vi "xyz-fluor_localisation.vi"(4 "Positive angle":dbl, 5 "Gy":dbl[][](array[numeric]), 6 "Gthr":dbl[][](array[numeric]), 7 "Gx":dbl[][](array[numeric]), 8 "R":dbl, 9 "weights":dbl[](array[numeric]), 10 "B points":dbl[][](array[numeric])=[[5.0, 3.0], [6.0, 6.0]], 11 "A points":dbl[][](array[numeric])=[[0.0, 1.0], [2.0, 3.0]]) -> (3 "XYZ":dbl[](array[numeric]))   [LabVIEW 2015]
doc: "INPUT\nR - radius of the window (should be >0.5)\nGx,Gy - horizontal and vertical local gradient images\nGthr - thresholded magnitude of local gradients (if not wired will be calculated from Gx,Gy)\nA points - 2xN array of first points that define lines\nB points - 2xN array of second points that define lines\nw - weights (1D array)\nPositive angle - angle in degrees that defines orientation of the image of the particle which corresponds to positive z-value\n\nOUTPUT\nXYZ - x,y position of the particle in pixels (for original image), z-value\n\nThis vi calculates XYZ position of the fluorescent particle in astigmatism based microscopy. XY is found as a least square intersection point of gradient lines. The image of local gradients (Gthr) is splitted into 4 parts: TOP, LEFT, BOTTOM, RIGHT, relative to the particle center (cx,cy). The least-square intersection of all gradient lines (Gx, Gy) is calculated for each part. These centers are forming two lines: TOP-BOTTOM and LEFT-RIGHT, which are called axes (similar to ellipses axes). The major of two axes represents the magnitude of the z-value. The sign of the z-value is determined according to the angPos value which should correspond to the position of the long axis of the elliptical image of the particle. angPos is not required to be accurate, however, setting it to ~45 degrees off the real angle will create sporadic change in the sign and, therefore, in z-value.\n\nAuthor: Anatolii Kashchuk"
panel:
  out "center":dbl[][](array[numeric])
  # "This vi finds centroid and z-value from the image of a particle\n\nAuthor: Anatolii Kashchuk"
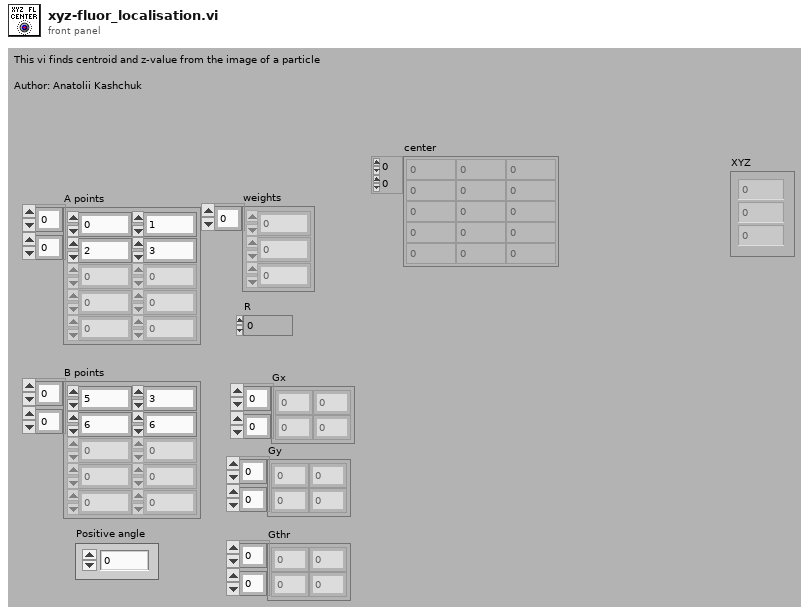
[diagram p1: front panel]
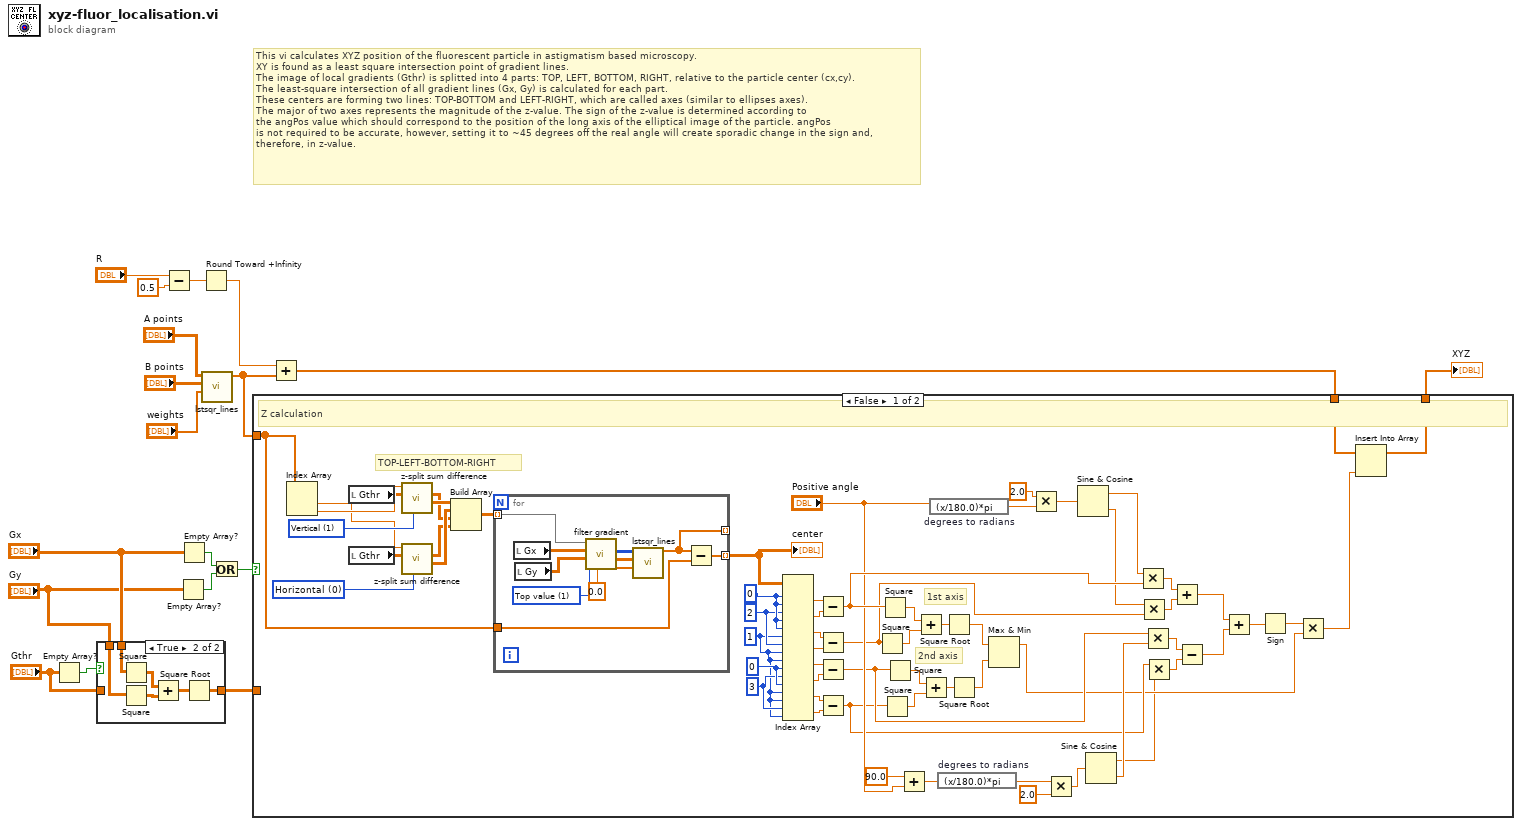
[diagram p0: block diagram]
diagram:
  # "This vi calculates XYZ position of the fluorescent particle in astigmatism based microscopy. \nXY is found as a least square intersection point of gradient lines. \nThe image of local gradients (Gthr) is splitted into 4 parts: TOP, LEFT, BOTTOM, RIGHT, relative to the particle center (cx,cy). \nThe least-square intersection of all gradient lines (Gx, Gy) is calculated for each part. \nThese centers are forming two lines: TOP-BOTTOM and LEFT-RIGHT, which are called axes (similar to ellipses axes). \nThe major of two axes represents the magnitude of the z-value. The sign of the z-value is determined according to \nthe angPos value which should correspond to the position of the long axis of the elliptical image of the particle. angPos\nis not required to be accurate, however, setting it to ~45 degrees off the real angle will create sporadic change in the sign and, \ntherefore, in z-value."
  n1 = Empty Array?(array="Gthr") -> (empty?=w6:bool)
  n2 = case shown="True" w6 {
    tunnel: "Gx" -> [_ w22]
    tunnel: "Gy" -> [_ w21]
    tunnel: [w19 w20] -> w3
    tunnel: "Gthr" -> [w19 _]
    frame False {
    }
    frame True {
      n3 = Square(x=w22) -> (x^2=w24:dbl[][])
      n4 = Square(x=w21) -> (x^2=w23:dbl[][])
      n5 = Add(x=w24, y=w23) -> (x+y=w25:dbl[][])
      n6 = Square Root(x=w25) -> (sqrt(x)=w20:dbl[][])
    }
  }
  n7 = Subtract(x="R", y=0.5) -> (x-y=w13:dbl)
  n8 = Empty Array?(array="Gy") -> (empty?=w7:bool)
  n9 = Empty Array?(array="Gx") -> (empty?=w8:bool)
  n10 = Round Toward +Infinity(x=w13) -> (ceil(x): smallest int >= x=w14:dbl)
  n11 = call "lstsqr_lines.vi"("weights"="weights", "B points"="B points", "A points"="A points") -> ("center"=w11:dbl[])  [unwired: 7 in, 1 out]
  n12 = Or(x=w8, y=w7) -> (x .or. y?=w1:bool)
  n13 = Add(x=w14, y=w11) -> (x+y=w10:dbl[])
  n14 = case shown="False" w1 {
    tunnel: w11 -> [w55 _]
    tunnel: w10 -> [w87 w100]
    tunnel: [w88 w100] -> w9
    tunnel: w3 -> [_ _]
    frame False {
      w64 = 3 ("disabled index (col)")
      w63 = 1 ("disabled index (col)")
      w71 = 2 ("index (row)")
      w65 = 0 ("disabled index (col)")
      w72 = 0 ("index (row)")
      w84 = u16 0 items=["Horizontal", "Vertical"] ("Text Ring")
      w86 = u16 1 items=["Horizontal", "Vertical"] ("Text Ring")
      # "2nd axis"
      # "X1\nX3\nY1\nY3\nX2\nX4\nY2\nY4"
      # "1st axis"
      # "TOP-LEFT-BOTTOM-RIGHT"
      # "Z calculation"
      n15 = Index Array(array=w55) -> (element #1=w83:dbl, element #2=w85:dbl)  [unwired: 2 in]
      n16 = local read "Gthr"() -> (w81:dbl[][])
      n17 = local read "Gthr"() -> (w82:dbl[][])
      n18 = call "z-split sum difference.vi"("split type"=w86, "G input"=w81, "center"=w85) -> ("left/top"=w80:dbl[][], "right/bottom"=w78:dbl[][])  [unwired: 6 in, 1 out]
      n19 = call "z-split sum difference.vi"("split type"=w84, "G input"=w82, "center"=w83) -> ("left/top"=w79:dbl[][], "right/bottom"=w77:dbl[][])  [unwired: 6 in, 1 out]
      n20 = Build Array(w80, w79, w78, w77) -> (w76:dbl[][][])
      n21 = for {
        tunnel: w76 -> [w99] mode=indexing
        tunnel: [w91] -> w75 mode=indexing
        tunnel: w55 -> [w90]
        tunnel: [w89] -> _ mode=indexing
        w95 = u16 1 items=["Top fraction", "Top value"] ("Threshold type")
        n22 = local read "Gx"() -> (w98:dbl[][])
        n23 = local read "Gy"() -> (w97:dbl[][])
        n24 = call "filter gradient.vi"("Threshold"=0.0, "Threshold type"=w95, "Gy"=w97, "Gx"=w98, "G"=w99) -> ("Weights"=w92:dbl[], "gradients"=w93:dbl[][], "centers"=w94:i32[][])  [unwired: 1 in, 3 out]
        n25 = call "lstsqr_lines.vi"("weights"=w92, "B points"=w93, "A points"=w94) -> ("center"=w89:dbl[])  [unwired: 7 in, 1 out]
        n26 = Subtract(x=w89, y=w90) -> (x-y=w91:dbl[])
      }
      "center" <- w75
      n27 = Index Array(array=w75, index (row) #1=w72, index (col) #1=w72, index (row) #2=w71, index (col) #2=w72, index (row) #3=w72, index (col) #3=w63, index (row) #4=w71, index (col) #4=w63, index (row) #5=w63, index (col) #5=w65, index (row) #6=w64, index (col) #6=w65, index (row) #7=w63, index (col) #7=w63, index (row) #8=w64, index (col) #8=w63) -> (element #1=w73:dbl, element #2=w74:dbl, element #3=w70:dbl, element #4=w69:dbl, element #5=w59:dbl, element #6=w58:dbl, element #7=w57:dbl, element #8=w56:dbl)
      n28 = Subtract(x=w73, y=w74) -> (x-y=w51:dbl)
      n29 = Subtract(x=w70, y=w69) -> (x-y=w42:dbl)
      n30 = Subtract(x=w59, y=w58) -> (x-y=w35:dbl)
      n31 = Subtract(x=w57, y=w56) -> (x-y=w33:dbl)
      n32 = Square(x=w42) -> (x^2=w67:dbl)
      n33 = Square(x=w51) -> (x^2=w68:dbl)
      n34 = Square(x=w33) -> (x^2=w61:dbl)
      n35 = Square(x=w35) -> (x^2=w60:dbl)
      n36 = Add(x=90.0, y="Positive angle") -> (x+y=w48:dbl)
      n37 = Add(x=w68, y=w67) -> (x+y=w66:dbl)
      n38 = Add(x=w60, y=w61) -> (x+y=w62:dbl)
      n39 = expression code="(x/180.0)*pi" "degrees to radians"("Positive angle") -> (w52:dbl)
      n40 = expression code="(x/180.0)*pi" "degrees to radians"(w48) -> (w46:dbl)
      n41 = Square Root(x=w66) -> (sqrt(x)=w54:dbl)
      n42 = Square Root(x=w62) -> (sqrt(x)=w53:dbl)
      n43 = Max & Min(x=w54, y=w53) -> (max(x,y)=w28:dbl)  [unwired: 1 out]
      n44 = Multiply(x=2.0 ("y"), y=w52) -> (x*y=w47:dbl)
      n45 = Multiply(x=w46, y=2.0) -> (x*y=w44:dbl)
      n46 = Sine & Cosine(0:w47) -> (1:w43:dbl, 2:w41:dbl)
      n47 = Sine & Cosine(0:w44) -> (1:w26:dbl, 2:w34:dbl)
      n48 = Multiply(x=w43, y=w51) -> (x*y=w40:dbl)
      n49 = Multiply(x=w41, y=w42) -> (x*y=w39:dbl)
      n50 = Multiply(x=w35, y=w34) -> (x*y=w37:dbl)
      n51 = Multiply(x=w33, y=w26) -> (x*y=w38:dbl)
      n52 = Add(x=w40, y=w39) -> (x+y=w32:dbl)
      n53 = Subtract(x=w37, y=w38) -> (x-y=w31:dbl)
      n54 = Add(x=w32, y=w31) -> (x+y=w30:dbl)
      n55 = Sign(1:w30) -> (0:w29:dbl)
      n56 = Multiply(x=w29, y=w28) -> (x*y=w27:dbl)
      n57 = Insert Into Array(array=w87, new element=w27) -> (w88:dbl[])  [unwired: 1 in]
    }
    frame True {
    }
  }
  "XYZ" <- w9
